vi "Set Trigger ID.vi"(10 "Trigger ID":u8, 11 "STS Process in":refnum<class "STS Process.lvclass">) -> (3 "STS Process out":refnum<class "STS Process.lvclass">)   [LabVIEW 2019, in "TimingDRV Engine.lvlib" / "STS Process.lvclass"]
uses:
  STS Process.lvclass
  STS Process.lvclass/STS Process.ctl
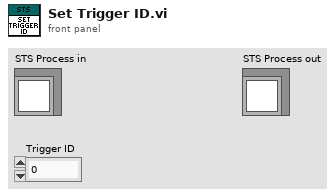
[diagram p1: front panel]
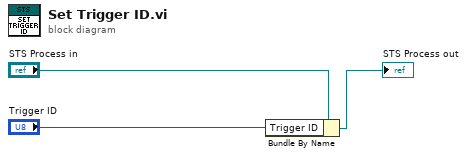
[diagram p0: block diagram]
diagram:
  n1 = Bundle By Name(cluster="STS Process in", "Trigger ID"="Trigger ID") -> (→"STS Process out":refnum<class "STS Process.lvclass">)
